vi "ImpedanceMatching.vi"() -> ()   [LabVIEW 2022 SP3]
panel:
  out "Lp (uH)":sgl
  out "Ls (uH)":dbl
  in  "Trans Xc":dbl
  in  "Q":dbl
  in  "Trans f":dbl
  in  "Transducer R":dbl
  out "L uH":dbl
  out "C2 pF":dbl
  out "C1 pF":dbl
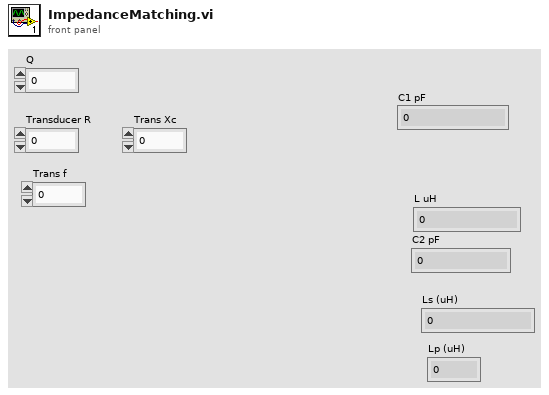
[diagram p1: front panel]
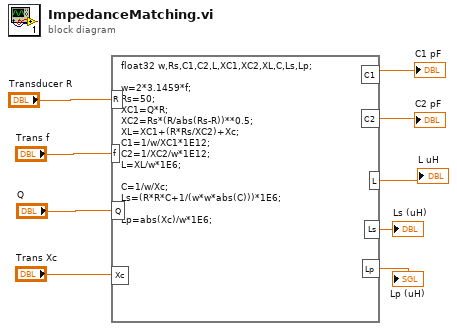
[diagram p0: block diagram]
diagram:
  n1 = formula code="float32 w,Rs,C1,C2,L,XC1,XC2,XL,C,Ls,Lp;\n\nw=2*3.1459*f;\nRs=50;\nXC1=Q*R;\nXC2=Rs*(R/abs(Rs-R))**0.5;\nXL=XC1+(R*Rs/XC2)+Xc;\nC1=1/w/XC1*1E12;\nC2=1/XC2/w*1E12;\nL=XL/w*1E6;\n\nC=1/w/Xc;\nLs=(R*R*C+1/(w*w*abs(C)))*1E6;\n\nLp=abs(Xc)/w*1E6;"("R"="Transducer R", "f"="Trans f", "Q"="Q", "Xc"="Trans Xc") -> ("C1"=→"C1 pF":sgl, "C2"=→"C2 pF":sgl, "L"=→"L uH":sgl, "Ls"=→"Ls (uH)":sgl, "Lp"=→"Lp (uH)":sgl)
